vi "CRYCurve Library Popup Menu.vi"(8 "Category?":bool, 9 "Group?":bool, 10 "Type":enum16{"Curves", "Values", "Results", "WFM"}(ring), 11 "Menu Ref In":refnum<k9>) -> (3 "Menu Ref Out":refnum<k9>)   [LabVIEW 2013]
uses:
  CRYMainGlobal.vi
  Global/CRYCurve Library Global.vi
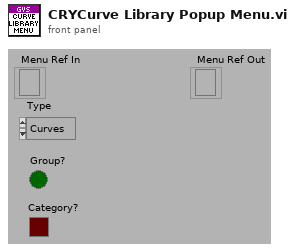
[diagram p1: front panel]
types:
  T1 = typedef "CRYCurveLib Info Cluster.ctl" = cluster{"GroupingState":string}
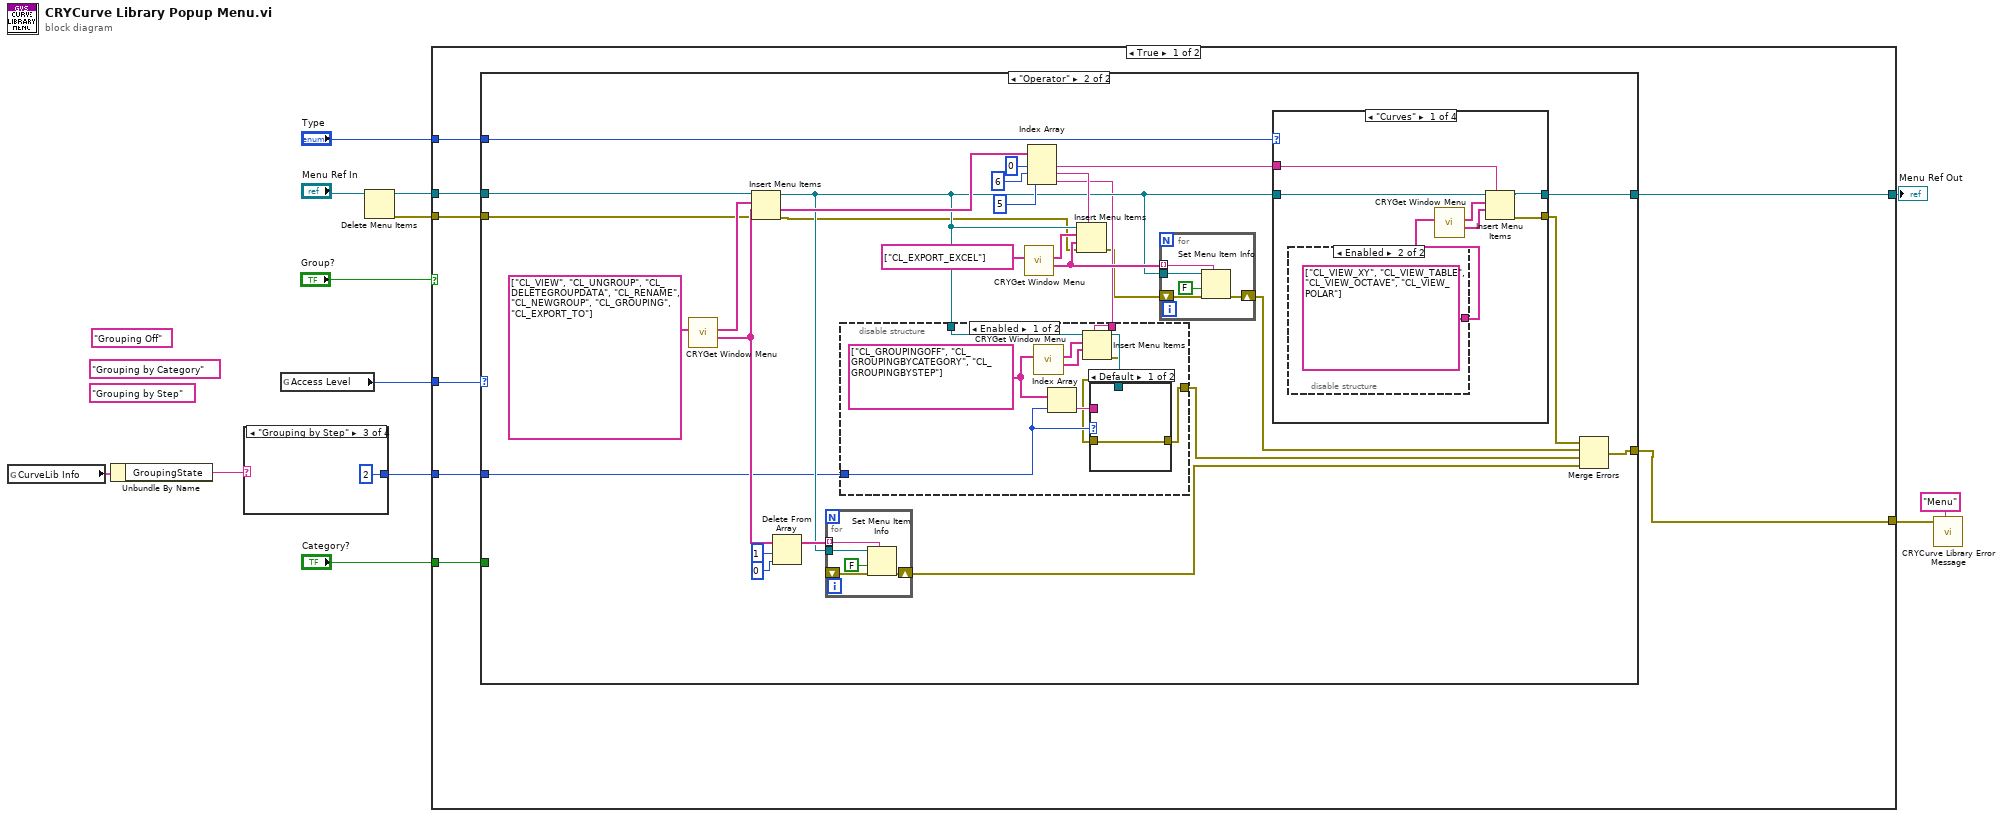
[diagram p0: block diagram]
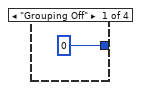
[diagram p2: hidden frame]
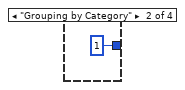
[diagram p3: hidden frame]
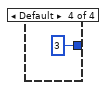
[diagram p4: hidden frame]
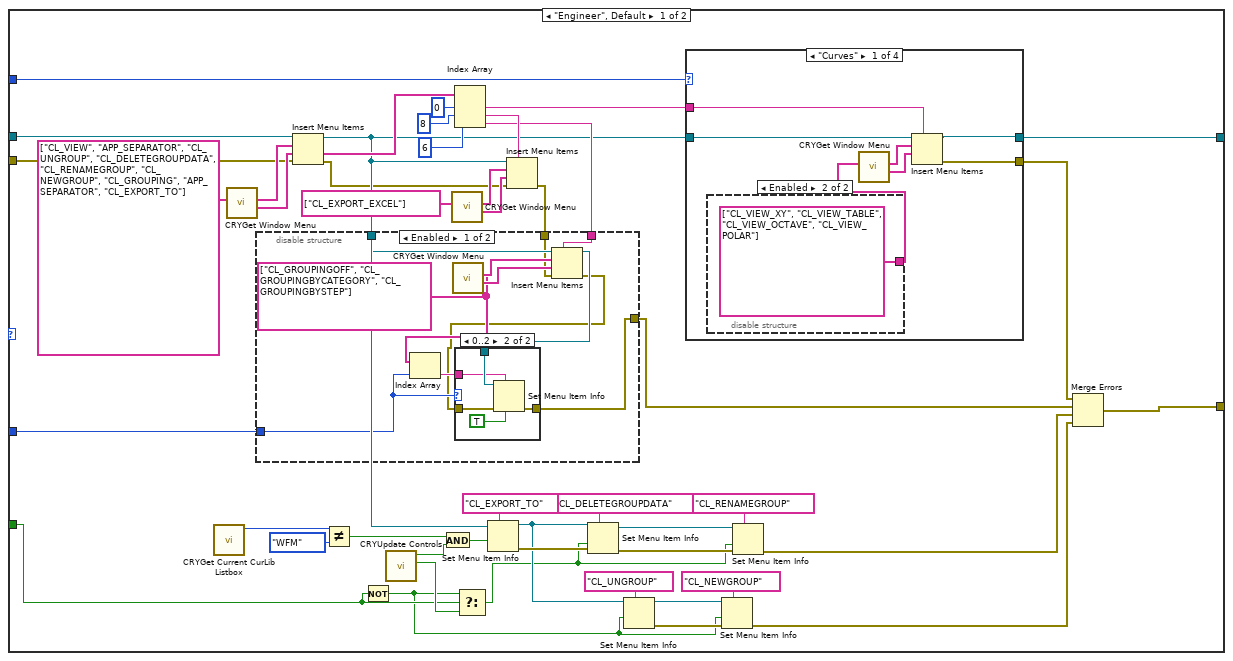
[diagram p5: hidden frame]
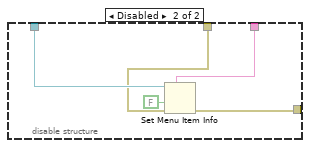
[diagram p7: hidden frame]
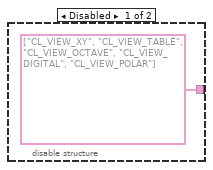
[diagram p8: hidden frame]
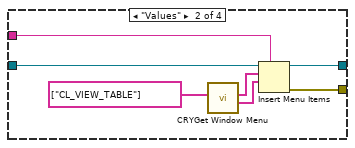
[diagram p9: hidden frame]
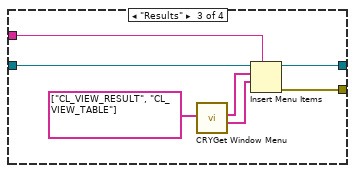
[diagram p10: hidden frame]
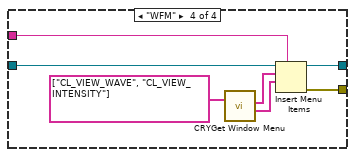
[diagram p11: hidden frame]
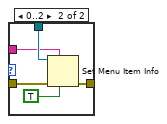
[diagram p12: hidden frame]
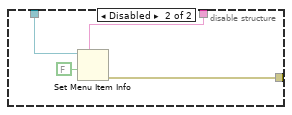
[diagram p13: hidden frame]
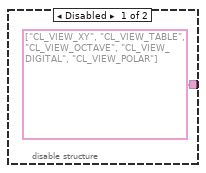
[diagram p14: hidden frame]
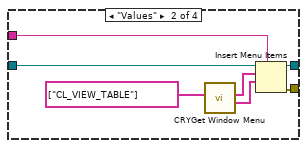
[diagram p15: hidden frame]
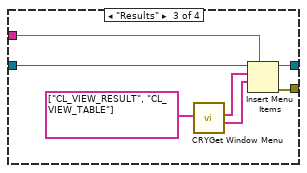
[diagram p16: hidden frame]
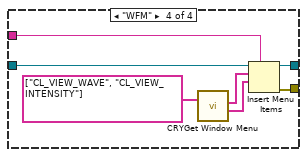
[diagram p17: hidden frame]
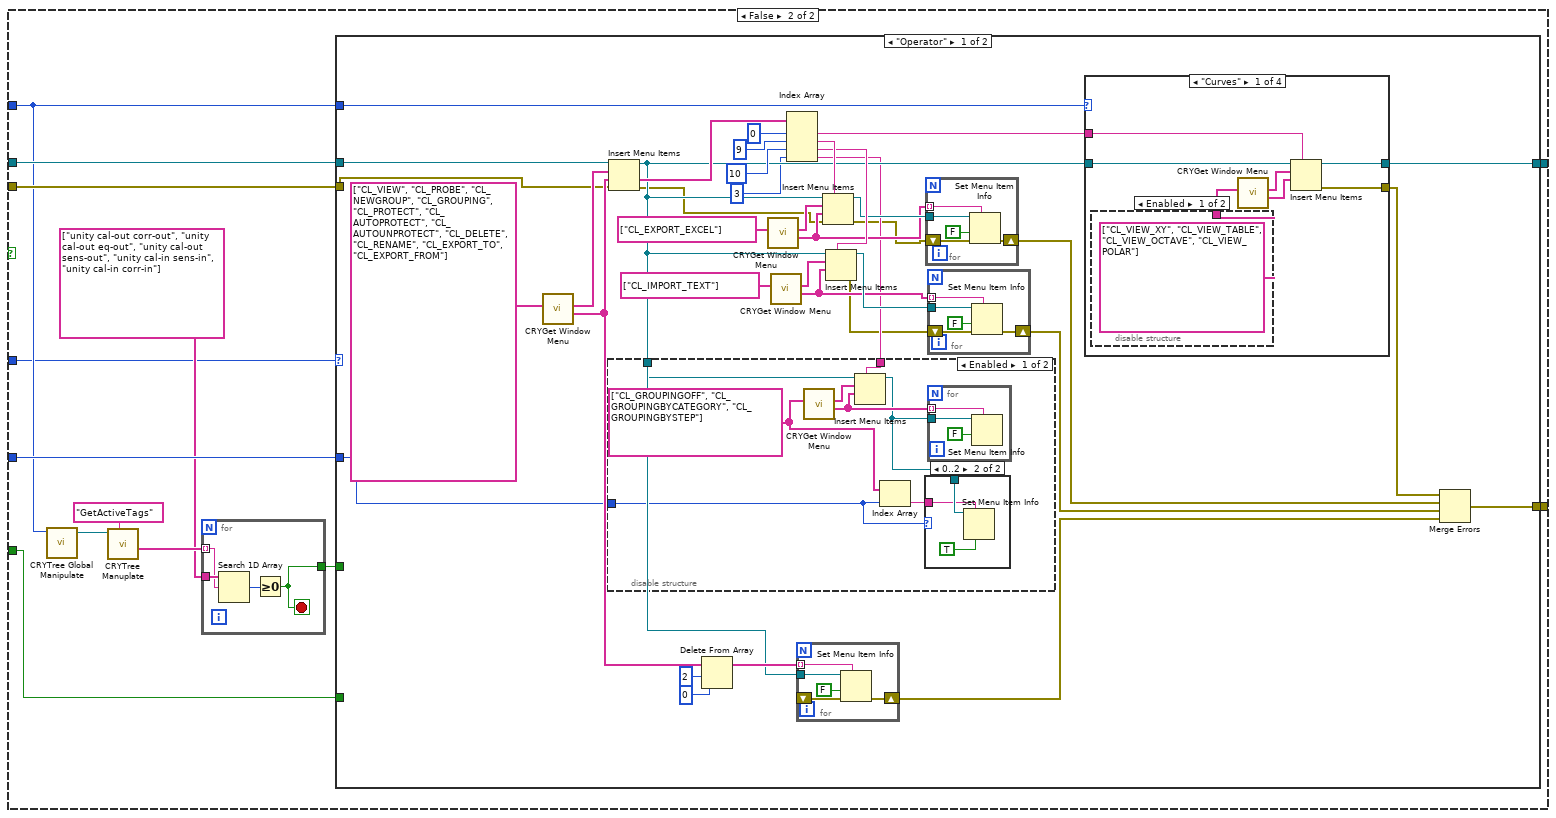
[diagram p18: hidden frame]
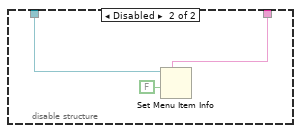
[diagram p20: hidden frame]
diagram:
  (unwired) "Grouping by Step" ("sAction")
  (unwired) "Grouping by Category" ("sAction")
  (unwired) "Grouping Off" ("sAction")
  n1 = global read "CRYCurve Library Global.vi" "CurveLib Info"() -> (w8:T1)
  n2 = Unbundle By Name(w8) -> ("GroupingState"=w7:string)
  n3 = case shown="\"Grouping by Step\"" w7 {
    tunnel: [0 ("length") 1 ("length") 2 ("length") 3 ("length")] -> w6
    frame "Grouping Off" {
    }
    frame "Grouping by Category" {
    }
    frame "Grouping by Step" {
    }
    frame Default {
    }
  }
  n4 = global read "CRYMainGlobal.vi" "Access Level"() -> (w1:enum16{"Engineer", "Technician", "Operator"})
  n5 = Delete Menu Items(9:"Menu Ref In") -> (0:w5:errorcluster, 3:w10:refnum<k9>)  [unwired: 2 in, 1 out]
  n6 = case shown="True" "Group?" {
    tunnel: "Type" -> [w25 w219]
    tunnel: [w24 w225] -> w11
    tunnel: w10 -> [w23 w220]
    tunnel: w1 -> [w22 w213]
    tunnel: w6 -> [w21 w224]
    tunnel: w5 -> [w20 w223]
    tunnel: [w19 w222] -> w4
    tunnel: "Category?" -> [w18 w214]
    frame True {
      n7 = case shown="\"Operator\"" w22 {
        tunnel: w25 -> [w71 w152]
        tunnel: [w70 w151] -> w24
        tunnel: w23 -> [w68 w149]
        tunnel: w21 -> [w45 w133]
        tunnel: w20 -> [w44 w131]
        tunnel: [w36 w124] -> w19
        tunnel: w18 -> [w27 _]
        frame "Engineer", Default {
          # "6"
          # "8"
          n8 = call "CRYGet Current CurLib Listbox.vi"() -> ("Type"=w51:enum16{"Curves", "Values", "Results", "WFM"})  [unwired: 9 in, 2 out]
          n9 = call "CRYGet Window Menu.vi"("Tags"=string[] ["CL_VIEW", "APP_SEPARATOR", "CL_UNGROUP", "CL_DELETEGROUPDATA", "CL_RENAMEGROUP", "CL_NEWGROUP", "CL_GROUPING", "APP_SEPARATOR", "CL_EXPORT_TO"] ("item tags")) -> ("Tags_Out"=w57:string[], "Names_Out"=w58:string[])  [unwired: 8 in, 1 out]
          n10 = Insert Menu Items(6:w44, 7:w57, 8:w58, 9:w68) -> (0:w43:errorcluster, 1:w69:string[], 3:w46:refnum<k9>)  [unwired: 2 out]
          n11 = Not Equal?(x=w51, y=enum16{"Curves", "Values", "Results", "WFM"}."WFM") -> (x != y?=w50:bool)
          n12 = Not(x=w27) -> (.not. x?=w26:bool)
          n13 = call "CRYUpdate Controls.vi"() -> ("Delete/Rename?"=w29:bool, "Save/Export?"=w49:bool)  [unwired: 1 in, 9 out]
          n14 = And(x=w50, y=w49) -> (x .and. y?=w52:bool)
          n15 = call "CRYGet Window Menu.vi"("Tags"=string[] ["CL_EXPORT_EXCEL"] ("item names")) -> ("Tags_Out"=w54:string[], "Names_Out"=w55:string[])  [unwired: 8 in, 1 out]
          n16 = Index Array(array=w69, index #1=0 ("index"), index #2=8 ("index"), index #3=6 ("index")) -> (element #1=w60:string, element #2=w62:string, element #3=w47:string)
          n17 = Select(t=w26, s=w27, f=w29) -> (s? t:f=w28:bool)
          n18 = Set Menu Item Info(7:"CL_EXPORT_TO", 9:w52, 11:w46) -> (0:w41:errorcluster, 3:w30:refnum<k9>)  [unwired: 1 in, 3 out]
          n19 = Insert Menu Items(5:w62, 6:w43, 7:w54, 8:w55, 9:w46) -> (0:w42:errorcluster)  [unwired: 3 out]
          n20 = disable-structure shown="Enabled" {
            disable-tunnel: w47 -> [w82 w92]
            disable-tunnel: w46 -> [w81 w93]
            disable-tunnel: w45 -> [w75 _]
            disable-tunnel: w42 -> [w74 w90]
            disable-tunnel: [w72 w89] -> w38
            frame Enabled {
              w76 = string[] ["CL_GROUPINGOFF", "CL_GROUPINGBYCATEGORY", "CL_GROUPINGBYSTEP"] ("item names")
              n21 = Index Array(array=w76, index=w75) -> (element=w78:string)
              n22 = call "CRYGet Window Menu.vi"("Tags"=w76) -> ("Tags_Out"=w79:string[], "Names_Out"=w80:string[])  [unwired: 8 in, 1 out]
              n23 = Insert Menu Items(5:w82, 6:w74, 7:w79, 8:w80, 9:w81) -> (0:w73:errorcluster, 3:w77:refnum<k9>)  [unwired: 2 out]
              n24 = case shown="0..2" w75 {
                tunnel: w77 -> [_ w88]
                tunnel: w78 -> [_ w87]
                tunnel: w73 -> [w83 w85]
                tunnel: [w83 w84] -> w72
                frame Default {
                }
                frame 0..2 {
                  n25 = Set Menu Item Info(6:TRUE ("checked"), 7:w87, 8:w85, 11:w88) -> (0:w84:errorcluster)  [unwired: 3 in, 1 out]
                }
              }
            }
            frame Disabled {
              n26 = Set Menu Item Info(7:w92, 8:w90, 9:FALSE ("checked"), 11:w93) -> (0:w89:errorcluster)  [unwired: 3 in, 1 out]
            }
          }
          n27 = Set Menu Item Info(7:"CL_DELETEGROUPDATA", 8:w41, 9:w28, 11:w30) -> (0:w40:errorcluster, 3:w65:refnum<k9>)  [unwired: 3 out]
          n28 = Set Menu Item Info(7:"CL_UNGROUP", 9:w26, 11:w30) -> (0:w33:errorcluster, 3:w31:refnum<k9>)  [unwired: 1 in, 3 out]
          n29 = case shown="\"Curves\"" w71 {
            tunnel: [w95 w107 w115 w122] -> w70
            tunnel: w46 -> [w100 w108 w116 w123]
            tunnel: w60 -> [w99 w109 w114 w121]
            tunnel: [w94 w103 w110 w117] -> w39
            frame "Curves" {
              n30 = disable-structure shown="Enabled" {
                disable-tunnel: [string[] ["CL_VIEW_XY", "CL_VIEW_TABLE", "CL_VIEW_OCTAVE", "CL_VIEW_DIGITAL", "CL_VIEW_POLAR"] ("item tags") string[] ["CL_VIEW_XY", "CL_VIEW_TABLE", "CL_VIEW_OCTAVE", "CL_VIEW_POLAR"] ("item tags")] -> w98
                frame Disabled {
                }
                frame Enabled {
                }
              }
              n31 = call "CRYGet Window Menu.vi"("Tags"=w98) -> ("Tags_Out"=w97:string[], "Names_Out"=w96:string[])  [unwired: 8 in, 1 out]
              n32 = Insert Menu Items(5:w99, 7:w97, 8:w96, 9:w100) -> (0:w94:errorcluster, 3:w95:refnum<k9>)  [unwired: 1 in, 2 out]
            }
            frame "Values" {
              n33 = call "CRYGet Window Menu.vi"("Tags"=string[] ["CL_VIEW_TABLE"] ("item tags")) -> ("Tags_Out"=w104:string[], "Names_Out"=w105:string[])  [unwired: 8 in, 1 out]
              n34 = Insert Menu Items(5:w109, 7:w104, 8:w105, 9:w108) -> (0:w103:errorcluster, 3:w107:refnum<k9>)  [unwired: 1 in, 2 out]
            }
            frame "Results" {
              n35 = call "CRYGet Window Menu.vi"("Tags"=string[] ["CL_VIEW_RESULT", "CL_VIEW_TABLE"] ("item tags")) -> ("Tags_Out"=w111:string[], "Names_Out"=w112:string[])  [unwired: 8 in, 1 out]
              n36 = Insert Menu Items(5:w114, 7:w111, 8:w112, 9:w116) -> (0:w110:errorcluster, 3:w115:refnum<k9>)  [unwired: 1 in, 2 out]
            }
            frame "WFM" {
              n37 = call "CRYGet Window Menu.vi"("Tags"=string[] ["CL_VIEW_WAVE", "CL_VIEW_INTENSITY"] ("item tags")) -> ("Tags_Out"=w118:string[], "Names_Out"=w119:string[])  [unwired: 8 in, 1 out]
              n38 = Insert Menu Items(5:w121, 7:w118, 8:w119, 9:w123) -> (0:w117:errorcluster, 3:w122:refnum<k9>)  [unwired: 1 in, 2 out]
            }
          }
          n39 = Set Menu Item Info(7:"CL_NEWGROUP", 8:w33, 9:w26, 11:w31) -> (0:w32:errorcluster)  [unwired: 4 out]
          n40 = Set Menu Item Info(7:"CL_RENAMEGROUP", 8:w40, 9:w28, 11:w65) -> (0:w37:errorcluster)  [unwired: 4 out]
          n41 = Merge Errors(w39, w38, w37, w32) -> (w36:errorcluster)
        }
        frame "Operator" {
          # "5"
          # "6"
          n42 = call "CRYGet Window Menu.vi"("Tags"=string[] ["CL_VIEW", "CL_UNGROUP", "CL_DELETEGROUPDATA", "CL_RENAME", "CL_NEWGROUP", "CL_GROUPING", "CL_EXPORT_TO"] ("item tags")) -> ("Tags_Out"=w138:string[], "Names_Out"=w143:string[])  [unwired: 8 in, 1 out]
          n43 = Insert Menu Items(6:w131, 7:w138, 8:w143, 9:w149) -> (0:w130:errorcluster, 1:w150:string[], 3:w134:refnum<k9>)  [unwired: 2 out]
          n44 = Delete From Array(array=w138, length=1, index=0) -> (array with subset deleted=w137:string[])  [unwired: 1 out]
          n45 = for {
            tunnel: w137 -> [w181] mode=indexing
            tunnel: w134 -> [w180]
            shift-right: [w179] -> w127
            shift-left: _ -> [w178]
            n46 = Set Menu Item Info(7:w181, 8:w178, 9:FALSE ("enabled"), 11:w180) -> (0:w179:errorcluster)  [unwired: 1 in, 3 out]
          }
          n47 = call "CRYGet Window Menu.vi"("Tags"=string[] ["CL_EXPORT_EXCEL"] ("item names")) -> ("Tags_Out"=w136:string[], "Names_Out"=w141:string[])  [unwired: 8 in, 1 out]
          n48 = Index Array(array=w150, index #1=0 ("index"), index #2=6 ("index"), index #3=5 ("index")) -> (element #1=w145:string, element #2=w147:string, element #3=w132:string)
          n49 = disable-structure shown="Enabled" {
            disable-tunnel: w134 -> [w160 w171]
            disable-tunnel: w133 -> [w156 _]
            disable-tunnel: w132 -> [w155 w170]
            disable-tunnel: [w153 w169] -> w126
            frame Enabled {
              w159 = string[] ["CL_GROUPINGOFF", "CL_GROUPINGBYCATEGORY", "CL_GROUPINGBYSTEP"] ("item names")
              n50 = call "CRYGet Window Menu.vi"("Tags"=w159) -> ("Tags_Out"=w161:string[], "Names_Out"=w162:string[])  [unwired: 8 in, 1 out]
              n51 = Index Array(array=w159, index=w156) -> (element=w157:string)
              n52 = Insert Menu Items(5:w155, 7:w161, 8:w162, 9:w160) -> (0:w154:errorcluster, 3:w158:refnum<k9>)  [unwired: 1 in, 2 out]
              n53 = case shown="Default" w156 {
                tunnel: w158 -> [_ w168]
                tunnel: w157 -> [_ w167]
                tunnel: w154 -> [w163 w165]
                tunnel: [w163 w164] -> w153
                frame Default {
                }
                frame 0..2 {
                  n54 = Set Menu Item Info(6:TRUE ("checked"), 7:w167, 8:w165, 11:w168) -> (0:w164:errorcluster)  [unwired: 3 in, 1 out]
                }
              }
            }
            frame Disabled {
              n55 = Set Menu Item Info(7:w170, 9:FALSE ("checked"), 11:w171) -> (0:w169:errorcluster)  [unwired: 4 in, 1 out]
            }
          }
          n56 = Insert Menu Items(5:w147, 6:w130, 7:w136, 8:w141, 9:w134) -> (0:w129:errorcluster)  [unwired: 3 out]
          n57 = for {
            tunnel: w136 -> [w176] mode=indexing
            tunnel: w134 -> [w175]
            shift-right: [w173] -> w128
            shift-left: w129 -> [w174]
            n58 = Set Menu Item Info(7:w176, 8:w174, 9:FALSE ("enabled"), 11:w175) -> (0:w173:errorcluster)  [unwired: 1 in, 3 out]
          }
          n59 = case shown="\"Curves\"" w152 {
            tunnel: [w184 w196 w204 w211] -> w151
            tunnel: w134 -> [w189 w197 w205 w212]
            tunnel: w145 -> [w188 w198 w203 w210]
            tunnel: [w183 w192 w199 w206] -> w125
            frame "Curves" {
              n60 = disable-structure shown="Enabled" {
                disable-tunnel: [string[] ["CL_VIEW_XY", "CL_VIEW_TABLE", "CL_VIEW_OCTAVE", "CL_VIEW_DIGITAL", "CL_VIEW_POLAR"] ("item tags") string[] ["CL_VIEW_XY", "CL_VIEW_TABLE", "CL_VIEW_OCTAVE", "CL_VIEW_POLAR"] ("item tags")] -> w187
                frame Disabled {
                }
                frame Enabled {
                }
              }
              n61 = call "CRYGet Window Menu.vi"("Tags"=w187) -> ("Tags_Out"=w186:string[], "Names_Out"=w185:string[])  [unwired: 8 in, 1 out]
              n62 = Insert Menu Items(5:w188, 7:w186, 8:w185, 9:w189) -> (0:w183:errorcluster, 3:w184:refnum<k9>)  [unwired: 1 in, 2 out]
            }
            frame "Values" {
              n63 = call "CRYGet Window Menu.vi"("Tags"=string[] ["CL_VIEW_TABLE"] ("item tags")) -> ("Tags_Out"=w193:string[], "Names_Out"=w194:string[])  [unwired: 8 in, 1 out]
              n64 = Insert Menu Items(5:w198, 7:w193, 8:w194, 9:w197) -> (0:w192:errorcluster, 3:w196:refnum<k9>)  [unwired: 1 in, 2 out]
            }
            frame "Results" {
              n65 = call "CRYGet Window Menu.vi"("Tags"=string[] ["CL_VIEW_RESULT", "CL_VIEW_TABLE"] ("item tags")) -> ("Tags_Out"=w200:string[], "Names_Out"=w201:string[])  [unwired: 8 in, 1 out]
              n66 = Insert Menu Items(5:w203, 7:w200, 8:w201, 9:w205) -> (0:w199:errorcluster, 3:w204:refnum<k9>)  [unwired: 1 in, 2 out]
            }
            frame "WFM" {
              n67 = call "CRYGet Window Menu.vi"("Tags"=string[] ["CL_VIEW_WAVE", "CL_VIEW_INTENSITY"] ("item tags")) -> ("Tags_Out"=w207:string[], "Names_Out"=w208:string[])  [unwired: 8 in, 1 out]
              n68 = Insert Menu Items(5:w210, 7:w207, 8:w208, 9:w212) -> (0:w206:errorcluster, 3:w211:refnum<k9>)  [unwired: 1 in, 2 out]
            }
          }
          n69 = Merge Errors(w125, w128, w126, w127) -> (w124:errorcluster)
        }
      }
    }
    frame False {
      n70 = call "CRYTree Global Manipulate.vi"("Type In"=w219) -> ("Tree/Curve Tree"=w218:refnum<vi>)  [unwired: 7 in, 3 out]
      n71 = call "CRYTree Manuplate.vi"("sAction"="GetActiveTags", "Tree in"=w218) -> ("sData Out"=w217:string[])  [unwired: 6 in, 3 out]
      n72 = for {
        tunnel: w217 -> [w228] mode=indexing
        tunnel: string[] ["unity cal-out corr-out", "unity cal-out eq-out", "unity cal-out sens-out", "unity cal-in sens-in", "unity cal-in corr-in"] ("item tags") -> [w229]
        tunnel: [w226] -> w215
        stop <- w226 stop-if-true
        n73 = Search 1D Array(1D array=w229, element=w228) -> (index of element=w227:i32)  [unwired: 1 in]
        n74 = Greater Or Equal To 0?(x=w227) -> (x >= 0?=w226:bool)
      }
      n75 = case shown="\"Operator\"" w213 {
        tunnel: w219 -> [w247 w403]
        tunnel: [w248 w402] -> w225
        tunnel: w220 -> [w256 w397]
        tunnel: w224 -> [w239 w360]
        tunnel: w223 -> [w238 w347]
        tunnel: [w230 w348] -> w222
        tunnel: w215 -> [_ w343]
        tunnel: w214 -> [_ w334]
        frame "Operator" {
          # "3"
          # "10"
          # "9"
          n76 = call "CRYGet Window Menu.vi"("Tags"=string[] ["CL_VIEW", "CL_PROBE", "CL_NEWGROUP", "CL_GROUPING", "CL_PROTECT", "CL_AUTOPROTECT", "CL_AUTOUNPROTECT", "CL_DELETE", "CL_RENAME", "CL_EXPORT_TO", "CL_EXPORT_FROM"] ("item tags")) -> ("Tags_Out"=w246:string[], "Names_Out"=w257:string[])  [unwired: 8 in, 1 out]
          n77 = Insert Menu Items(6:w238, 7:w246, 8:w257, 9:w256) -> (0:w237:errorcluster, 1:w266:string[], 3:w242:refnum<k9>)  [unwired: 2 out]
          n78 = Delete From Array(array=w246, length=2, index=0) -> (array with subset deleted=w243:string[])  [unwired: 1 out]
          n79 = call "CRYGet Window Menu.vi"("Tags"=string[] ["CL_EXPORT_EXCEL"] ("item names")) -> ("Tags_Out"=w252:string[], "Names_Out"=w253:string[])  [unwired: 8 in, 1 out]
          n80 = call "CRYGet Window Menu.vi"("Tags"=string[] ["CL_IMPORT_TEXT"] ("item names")) -> ("Tags_Out"=w251:string[], "Names_Out"=w250:string[])  [unwired: 8 in, 1 out]
          n81 = Index Array(array=w266, index #1=0 ("index"), index #2=9 ("index"), index #3=10 ("index"), index #4=3 ("index")) -> (element #1=w249:string, element #2=w264:string, element #3=w258:string, element #4=w240:string)
          n82 = disable-structure shown="Enabled" {
            disable-tunnel: w242 -> [w273 w282]
            disable-tunnel: w240 -> [w271 w281]
            disable-tunnel: w239 -> [w267 _]
            frame Enabled {
              w268 = string[] ["CL_GROUPINGOFF", "CL_GROUPINGBYCATEGORY", "CL_GROUPINGBYSTEP"] ("item names")
              n83 = call "CRYGet Window Menu.vi"("Tags"=w268) -> ("Tags_Out"=w272:string[], "Names_Out"=w274:string[])  [unwired: 8 in, 1 out]
              n84 = Insert Menu Items(5:w271, 7:w272, 8:w274, 9:w273) -> (3:w269:refnum<k9>)  [unwired: 1 in, 3 out]
              n85 = Index Array(array=w268, index=w267) -> (element=w270:string)
              n86 = case shown="0..2" w267 {
                tunnel: w269 -> [_ w277]
                tunnel: w270 -> [_ w276]
                frame Default {
                }
                frame 0..2 {
                  n87 = Set Menu Item Info(6:TRUE ("checked"), 7:w276, 11:w277) -> ()  [unwired: 4 in, 2 out]
                }
              }
              n88 = for {
                tunnel: w272 -> [w280] mode=indexing
                tunnel: w269 -> [w279]
                n89 = Set Menu Item Info(7:w280, 9:FALSE ("enabled"), 11:w279) -> ()  [unwired: 2 in, 4 out]
              }
            }
            frame Disabled {
              n90 = Set Menu Item Info(7:w281, 9:FALSE ("checked"), 11:w282) -> ()  [unwired: 4 in, 2 out]
            }
          }
          n91 = for {
            tunnel: w243 -> [w328] mode=indexing
            tunnel: w242 -> [w327]
            shift-right: [w325] -> w231
            shift-left: _ -> [w324]
            n92 = Set Menu Item Info(7:w328, 8:w324, 9:FALSE ("enabled"), 11:w327) -> (0:w325:errorcluster)  [unwired: 1 in, 3 out]
          }
          n93 = Insert Menu Items(5:w264, 6:w237, 7:w252, 8:w253, 9:w242) -> (0:w236:errorcluster, 3:w255:refnum<k9>)  [unwired: 2 out]
          n94 = Insert Menu Items(5:w258, 7:w251, 8:w250, 9:w242) -> (0:w235:errorcluster, 3:w254:refnum<k9>)  [unwired: 1 in, 2 out]
          n95 = for {
            tunnel: w252 -> [w323] mode=indexing
            tunnel: w255 -> [w322]
            shift-right: [w320] -> w233
            shift-left: w236 -> [w319]
            n96 = Set Menu Item Info(7:w323, 8:w319, 9:FALSE ("enabled"), 11:w322) -> (0:w320:errorcluster)  [unwired: 1 in, 3 out]
          }
          n97 = for {
            tunnel: w251 -> [w318] mode=indexing
            tunnel: w254 -> [w317]
            shift-right: [w315] -> w232
            shift-left: w235 -> [w314]
            n98 = Set Menu Item Info(7:w318, 8:w314, 9:FALSE ("enabled"), 11:w317) -> (0:w315:errorcluster)  [unwired: 1 in, 3 out]
          }
          n99 = case shown="\"Curves\"" w247 {
            tunnel: [w288 w297 w305 w312] -> w248
            tunnel: w242 -> [w290 w298 w306 w313]
            tunnel: w249 -> [w289 w299 w304 w311]
            tunnel: [w284 w293 w300 w307] -> w234
            frame "Curves" {
              n100 = disable-structure shown="Enabled" {
                disable-tunnel: [string[] ["CL_VIEW_XY", "CL_VIEW_TABLE", "CL_VIEW_OCTAVE", "CL_VIEW_POLAR"] ("item tags") string[] ["CL_VIEW_XY", "CL_VIEW_TABLE", "CL_VIEW_OCTAVE", "CL_VIEW_DIGITAL", "CL_VIEW_POLAR"] ("item tags")] -> w287
                frame Enabled {
                }
                frame Disabled {
                }
              }
              n101 = call "CRYGet Window Menu.vi"("Tags"=w287) -> ("Tags_Out"=w286:string[], "Names_Out"=w285:string[])  [unwired: 8 in, 1 out]
              n102 = Insert Menu Items(5:w289, 7:w286, 8:w285, 9:w290) -> (0:w284:errorcluster, 3:w288:refnum<k9>)  [unwired: 1 in, 2 out]
            }
            frame "Values" {
              n103 = call "CRYGet Window Menu.vi"("Tags"=string[] ["CL_VIEW_TABLE"] ("item tags")) -> ("Tags_Out"=w294:string[], "Names_Out"=w295:string[])  [unwired: 8 in, 1 out]
              n104 = Insert Menu Items(5:w299, 7:w294, 8:w295, 9:w298) -> (0:w293:errorcluster, 3:w297:refnum<k9>)  [unwired: 1 in, 2 out]
            }
            frame "Results" {
              n105 = call "CRYGet Window Menu.vi"("Tags"=string[] ["CL_VIEW_RESULT", "CL_VIEW_TABLE"] ("item tags")) -> ("Tags_Out"=w301:string[], "Names_Out"=w302:string[])  [unwired: 8 in, 1 out]
              n106 = Insert Menu Items(5:w304, 7:w301, 8:w302, 9:w306) -> (0:w300:errorcluster, 3:w305:refnum<k9>)  [unwired: 1 in, 2 out]
            }
            frame "WFM" {
              n107 = call "CRYGet Window Menu.vi"("Tags"=string[] ["CL_VIEW_WAVE", "CL_VIEW_INTENSITY"] ("item tags")) -> ("Tags_Out"=w308:string[], "Names_Out"=w309:string[])  [unwired: 8 in, 1 out]
              n108 = Insert Menu Items(5:w311, 7:w308, 8:w309, 9:w313) -> (0:w307:errorcluster, 3:w312:refnum<k9>)  [unwired: 1 in, 2 out]
            }
          }
          n109 = Merge Errors(w234, w233, w232, w231) -> (w230:errorcluster)
        }
        frame "Engineer", Default {
          # "4"
          # "13"
          # "14"
          n110 = call "CRYGet Current CurLib Listbox.vi"() -> ("Type"=w368:enum16{"Curves", "Values", "Results", "WFM"})  [unwired: 9 in, 2 out]
          n111 = call "CRYGet Window Menu.vi"("Tags"=string[] ["CL_VIEW", "CL_PROBE", "APP_SEPARATOR", "CL_NEWGROUP", "CL_GROUPING", "APP_SEPARATOR", "CL_PROTECT", "CL_AUTOPROTECT", "CL_AUTOUNPROTECT", "APP_SEPARATOR", "CL_DELETE", "CL_RENAME", "APP_SEPARATOR", "CL_EXPORT_TO", "CL_EXPORT_FROM"] ("item tags")) -> ("Tags_Out"=w381:string[], "Names_Out"=w382:string[])  [unwired: 8 in, 1 out]
          n112 = Insert Menu Items(6:w347, 7:w381, 8:w382, 9:w397) -> (0:w359:errorcluster, 1:w398:string[], 3:w344:refnum<k9>)  [unwired: 2 out]
          n113 = Not(x=w343) -> (.not. x?=w342:bool)
          n114 = Not Equal?(x=w368, y=enum16{"Curves", "Values", "Results", "WFM"}."Results") -> (x != y?=w365:bool)
          n115 = Not Equal?(x=w368, y=enum16{"Curves", "Values", "Results", "WFM"}."WFM") -> (x != y?=w367:bool)
          n116 = call "CRYUpdate Controls.vi"() -> ("Protect?"=w401:bool, "Delete/Rename?"=w370:bool, "AutoProtect?"=w400:bool, "Import?"=w366:bool, "UndoAutoProtect?"=w399:bool)  [unwired: 1 in, 6 out]
          n117 = And(x=w367, y=w365) -> (x .and. y?=w364:bool)
          n118 = And(x=w367, y=w370) -> (x .and. y?=w371:bool)
          n119 = call "CRYGet Window Menu.vi"("Tags"=string[] ["CL_EXPORT_EXCEL"] ("item names")) -> ("Tags_Out"=w378:string[], "Names_Out"=w379:string[])  [unwired: 8 in, 1 out]
          n120 = call "CRYGet Window Menu.vi"("Tags"=string[] ["CL_IMPORT_TEXT"] ("item names")) -> ("Tags_Out"=w375:string[], "Names_Out"=w374:string[])  [unwired: 8 in, 1 out]
          n121 = And(x=w366, y=w364) -> (x .and. y?=w363:bool)
          n122 = Index Array(array=w398, index #1=0 ("index"), index #2=13 ("index"), index #3=14 ("index"), index #4=4 ("index")) -> (element #1=w384:string, element #2=w386:string, element #3=w346:string, element #4=w361:string)
          n123 = disable-structure shown="Enabled" {
            disable-tunnel: w344 -> [w411 w422]
            disable-tunnel: w361 -> [w410 w421]
            disable-tunnel: w360 -> [w406 _]
            disable-tunnel: [w404 w420] -> w352
            frame Enabled {
              w407 = string[] ["CL_GROUPINGOFF", "CL_GROUPINGBYCATEGORY", "CL_GROUPINGBYSTEP"] ("item names")
              n124 = call "CRYGet Window Menu.vi"("Tags"=w407) -> ("Tags_Out"=w412:string[], "Names_Out"=w413:string[])  [unwired: 8 in, 1 out]
              n125 = Index Array(array=w407, index=w406) -> (element=w409:string)
              n126 = Insert Menu Items(5:w410, 7:w412, 8:w413, 9:w411) -> (0:w405:errorcluster, 3:w408:refnum<k9>)  [unwired: 1 in, 2 out]
              n127 = case shown="0..2" w406 {
                tunnel: w408 -> [_ w419]
                tunnel: w409 -> [_ w418]
                tunnel: w405 -> [w414 w416]
                tunnel: [w414 w415] -> w404
                frame Default {
                }
                frame 0..2 {
                  n128 = Set Menu Item Info(6:TRUE ("checked"), 7:w418, 8:w416, 11:w419) -> (0:w415:errorcluster)  [unwired: 3 in, 1 out]
                }
              }
            }
            frame Disabled {
              n129 = Set Menu Item Info(7:w421, 9:FALSE ("checked"), 11:w422) -> (0:w420:errorcluster)  [unwired: 4 in, 1 out]
            }
          }
          n130 = Set Menu Item Info(7:"CL_EXPORT_TO", 9:w371, 11:w344) -> (0:w358:errorcluster, 3:w391:refnum<k9>)  [unwired: 1 in, 3 out]
          n131 = Set Menu Item Info(7:"CL_EXPORT_FROM", 9:w363, 11:w344) -> (0:w336:errorcluster, 3:w335:refnum<k9>)  [unwired: 1 in, 3 out]
          n132 = Insert Menu Items(5:w386, 6:w359, 7:w378, 8:w379, 9:w344) -> (0:w354:errorcluster)  [unwired: 3 out]
          n133 = Insert Menu Items(5:w346, 7:w375, 8:w374, 9:w344) -> (0:w353:errorcluster, 1:w341:string[])  [unwired: 1 in, 2 out]
          n134 = Index Array(array=w341) -> (element=w340:string)  [unwired: 1 in]
          n135 = Set Menu Item Info(7:w340, 9:w342, 11:w344) -> (0:w345:errorcluster)  [unwired: 4 in, 1 out]
          n136 = Not(x=w334) -> (.not. x?=w333:bool)
          n137 = Set Menu Item Info(7:"CL_DELETE", 8:w358, 9:w370, 11:w391) -> (0:w357:errorcluster, 3:w338:refnum<k9>)  [unwired: 1 in, 2 out]
          n138 = Set Menu Item Info(7:"CL_RENAME", 8:w357, 9:w370, 11:w338) -> (0:w356:errorcluster, 3:w393:refnum<k9>)  [unwired: 3 out]
          n139 = Merge Errors(w354, w353, w352, w345) -> (w351:errorcluster)
          n140 = Select(t=w333, s=w334, f=TRUE) -> (s? t:f=w331:bool)
          n141 = Set Menu Item Info(7:"CL_PROTECT", 8:w356, 9:w401, 11:w393) -> (0:w329:errorcluster, 3:w330:refnum<k9>)  [unwired: 3 out]
          n142 = Set Menu Item Info(7:"CL_NEWGROUP", 8:w336, 9:w331, 11:w335) -> (0:w337:errorcluster)  [unwired: 4 out]
          n143 = case shown="\"Curves\"" w403 {
            tunnel: [w425 w437 w445 w452] -> w402
            tunnel: w344 -> [w430 w438 w446 w453]
            tunnel: w384 -> [w429 w439 w444 w451]
            tunnel: [w424 w433 w440 w447] -> w350
            frame "Curves" {
              n144 = disable-structure shown="Enabled" {
                disable-tunnel: [string[] ["CL_VIEW_XY", "CL_VIEW_TABLE", "CL_VIEW_OCTAVE", "CL_VIEW_DIGITAL", "CL_VIEW_POLAR"] ("item tags") string[] ["CL_VIEW_XY", "CL_VIEW_TABLE", "CL_VIEW_OCTAVE", "CL_VIEW_POLAR"] ("item tags")] -> w428
                frame Disabled {
                }
                frame Enabled {
                }
              }
              n145 = call "CRYGet Window Menu.vi"("Tags"=w428) -> ("Tags_Out"=w427:string[], "Names_Out"=w426:string[])  [unwired: 8 in, 1 out]
              n146 = Insert Menu Items(5:w429, 7:w427, 8:w426, 9:w430) -> (0:w424:errorcluster, 3:w425:refnum<k9>)  [unwired: 1 in, 2 out]
            }
            frame "Values" {
              n147 = call "CRYGet Window Menu.vi"("Tags"=string[] ["CL_VIEW_TABLE"] ("item tags")) -> ("Tags_Out"=w434:string[], "Names_Out"=w435:string[])  [unwired: 8 in, 1 out]
              n148 = Insert Menu Items(5:w439, 7:w434, 8:w435, 9:w438) -> (0:w433:errorcluster, 3:w437:refnum<k9>)  [unwired: 1 in, 2 out]
            }
            frame "Results" {
              n149 = call "CRYGet Window Menu.vi"("Tags"=string[] ["CL_VIEW_RESULT", "CL_VIEW_TABLE"] ("item tags")) -> ("Tags_Out"=w441:string[], "Names_Out"=w442:string[])  [unwired: 8 in, 1 out]
              n150 = Insert Menu Items(5:w444, 7:w441, 8:w442, 9:w446) -> (0:w440:errorcluster, 3:w445:refnum<k9>)  [unwired: 1 in, 2 out]
            }
            frame "WFM" {
              n151 = call "CRYGet Window Menu.vi"("Tags"=string[] ["CL_VIEW_WAVE", "CL_VIEW_INTENSITY"] ("item tags")) -> ("Tags_Out"=w448:string[], "Names_Out"=w449:string[])  [unwired: 8 in, 1 out]
              n152 = Insert Menu Items(5:w451, 7:w448, 8:w449, 9:w453) -> (0:w447:errorcluster, 3:w452:refnum<k9>)  [unwired: 1 in, 2 out]
            }
          }
          n153 = Set Menu Item Info(7:"CL_AUTOPROTECT", 8:w329, 9:w400, 11:w330) -> (0:w355:errorcluster, 3:w389:refnum<k9>)  [unwired: 3 out]
          n154 = Set Menu Item Info(7:"CL_AUTOUNPROTECT", 8:w355, 9:w399, 11:w389) -> (0:w349:errorcluster)  [unwired: 4 out]
          n155 = Merge Errors(w350, w351, w349, w337) -> (w348:errorcluster)
        }
      }
    }
  }
  "Menu Ref Out" <- w11
  n156 = call "CRYCurve Library Error Message.vi"("sAction"="Menu", "error IO"=w4) -> ()  [unwired: 10 in]
